vi "save_xy_cluster.vi"(9 "error in":errorcluster, 11 "Array":cluster{dbl, dbl}[](array[cluster])) -> (1 "error out":errorcluster)   [LabVIEW 2023]
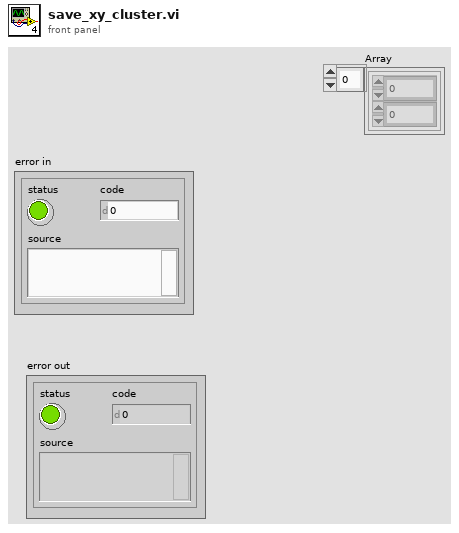
[diagram p1: front panel]
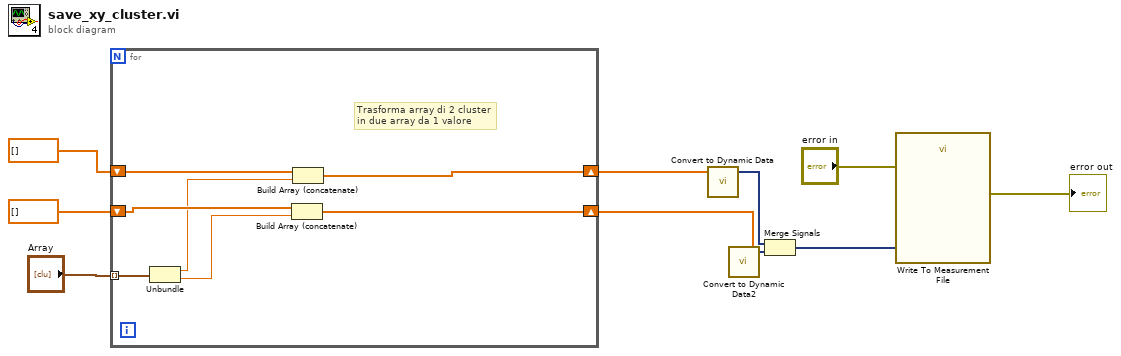
[diagram p0: block diagram]
diagram:
  n1 = for {
    shift-right: [w15] -> w7
    shift-left: dbl[] [] -> [w17]
    shift-right: [w14] -> w4
    shift-left: dbl[] [] -> [w16]
    tunnel: "Array" -> [w13] mode=indexing
    # "Trasforma array di 2 cluster\nin due array da 1 valore"
    n2 = Unbundle(w13) -> (w12:dbl, w11:dbl)
    n3 = Build Array (concatenate)(w16, w11) -> (w14:dbl[])
    n4 = Build Array (concatenate)(w17, w12) -> (w15:dbl[])
  }
  n5 = call "Convert to Dynamic Data"("Array"=w7) -> ("Dynamic Data Type"=w6:dynamicdata)  [unwired: 3 in]
  n6 = call "Convert to Dynamic Data2"("Array"=w4) -> ("Dynamic Data Type"=w3:dynamicdata)  [unwired: 3 in]
  n7 = Merge Signals(w6, w3) -> (w5:dynamicdata)
  n8 = call "Write To Measurement File"("Signals"=w5, "error in (no error)"="error in") -> ("error out"=→"error out":errorcluster)  [unwired: 15 in, 2 out]
